vi "Write Notifier Ref.vi"(8 "error in":errorcluster, 10 "Notifier Ref":refnum<notifier>, 11 "NotifierMessageTransport in":refnum<class "NotifierMessageTransport.lvclass">) -> (0 "error out":errorcluster, 3 "NotifierMessageTransport out":refnum<class "NotifierMessageTransport.lvclass">)   [LabVIEW 2016, in "NotifierMessageTransport.lvclass"]
uses:
  NotifierMessageTransport.lvclass
  IMessagePayload/IMessagePayload.lvclass
  NotifierMessageTransport.lvclass/NotifierMessageTransport.ctl
panel:
  # "INPUTS"
  # "OUTPUTS"
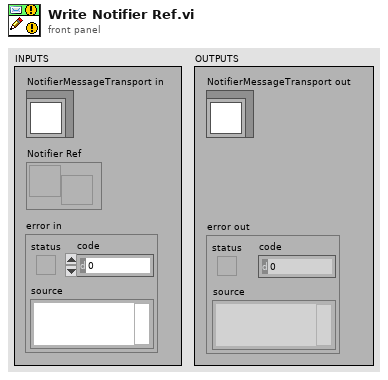
[diagram p1: front panel]
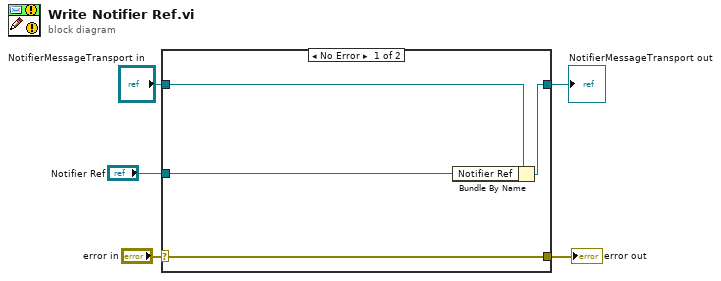
[diagram p0: block diagram]
diagram:
  n1 = case shown="No Error" "error in" {
    selector: "error in" -> [w9 w10]
    tunnel: [w9 w10] -> w4
    tunnel: [w7 w11] -> w2
    tunnel: "NotifierMessageTransport in" -> [w8 w11]
    tunnel: "Notifier Ref" -> [w6 _]
    frame No Error {
      n2 = Bundle By Name(cluster=w8, "Notifier Ref"=w6) -> (w7:refnum<class "NotifierMessageTransport.lvclass">)
    }
    frame Error {
    }
  }
  "error out" <- w4
  "NotifierMessageTransport out" <- w2
